vi "Add Clients.vi"(8 "error in (no error)":errorcluster, 9 "End Point Queue":refnum<class "Message Queue.lvclass">, 10 "Client":string, 11 "Server Client in":refnum<class "Server Client.lvclass">) -> (0 "error out":errorcluster, 3 "Server Client out":refnum<class "Server Client.lvclass">)   [LabVIEW 2020, in "Server Client.lvclass"]
uses:
  Server Client.lvclass
  <vilib>/addons/_Workers/Library/Classes/Message Queue/Message Queue.lvclass
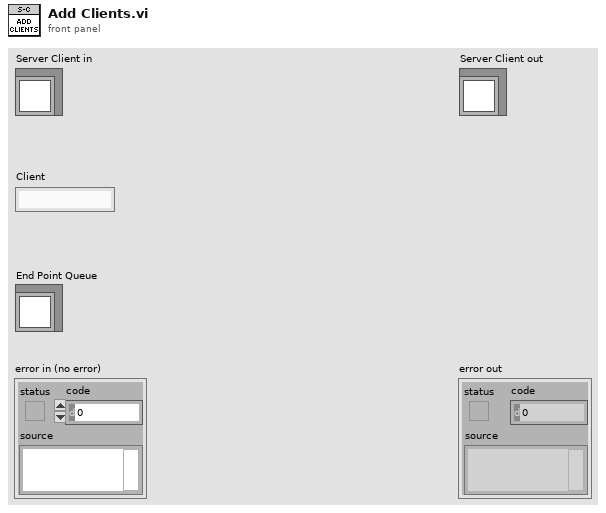
[diagram p1: front panel]
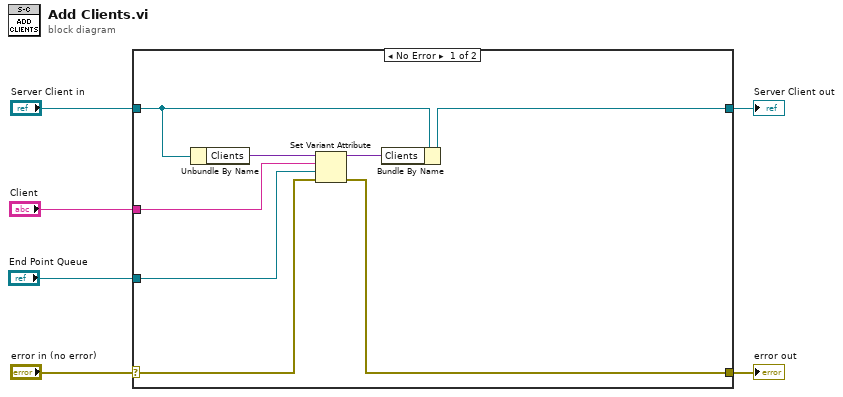
[diagram p0: block diagram]
diagram:
  n1 = case shown="No Error" "error in (no error)" {
    selector: "error in (no error)" -> [w10 w16]
    tunnel: [w7 w16] -> w5
    tunnel: [w9 w15] -> w3
    tunnel: "Server Client in" -> [w14 w15]
    tunnel: "Client" -> [w12 _]
    tunnel: "End Point Queue" -> [w11 _]
    frame No Error {
      n2 = Unbundle By Name(w14) -> ("Clients"=w13:variant)
      n3 = Set Variant Attribute(Variant=w13, name=w12, value=w11, error in=w10) -> (Variant out=w8:variant, error out=w7:errorcluster)  [unwired: 1 out]
      n4 = Bundle By Name(cluster=w14, "Clients"=w8) -> (w9:refnum<class "Server Client.lvclass">)
    }
    frame Error {
    }
  }
  "error out" <- w5
  "Server Client out" <- w3
